vi "2-1三角函数实现(notcomplete).vi"() -> ()   [LabVIEW 2018]
uses:
  <vilib>/Analysis/3filter.llb/Filter Passband Type.ctl
  <vilib>/Analysis/3filter.llb/Butterworth Filter (DBL).vi
  <vilib>/express/express analysis/Spectral/Block/exnSpectralBlock spectral measurements peak poly.vi
  <vilib>/express/express analysis/Spectral/Block/exnSpectralBlock spectral measurements peak WFM.vi
  <vilib>/express/express analysis/Spectral/XNode/ExpressSpectralMeasurementsBlockNode.xnode
  <vilib>/measure/NI_MABase.lvlib
  <vilib>/Analysis/NI_AALBase.lvlib
  <vilib>/Analysis/NI_AALPro.lvlib
panel:
  out "载波信号":waveform(dbl)(graph)
  out "β":dbl
  in  "选项卡控件":enum32{"调制", "滤波", "解调"}(tab)
  out "频域":cluster{"f0":dbl, "df":dbl, "magnitude":dbl[]}(graph)
  out "时域":waveform(dbl)[](graph)
  out "频域":cluster{"f0":dbl, "df":dbl, "magnitude":dbl[]}(graph)
  out "时域":waveform(dbl)(graph)
  out "时域 2":waveform(dbl)(graph)
  in  "带通Butterworth滤波器":cluster{"中心频率(Hz)":dbl, "带宽(Hz)":dbl}={"中心频率(Hz)"=150000.0, "带宽(Hz)"=30000.0}
  out "BT(Hz)":dbl
  out "调制信号":waveform(dbl)(graph)
  out "采样参数（采样频率fs，采样数Ns）":cluster{dbl, dbl} {"?" format="%#_6f"; "?" format="%#_6f"}
  in  "kf(Hz/V)":dbl=50000.0
  in  "An(V)":dbl=0.02
  in  "调制信号":cluster{"fm(Hz)":dbl, "Am(V)":dbl}={"fm(Hz)"=5000.0, "Am(V)"=1.0}
  in  "载波信号":cluster{"fc(Hz)":dbl, "Ac(V)":dbl}={"fc(Hz)"=150000.0, "Ac(V)"=1.0}
  # "要显示n个周期的调制信号波形，\n则采样数Ns=n*fs/fm"
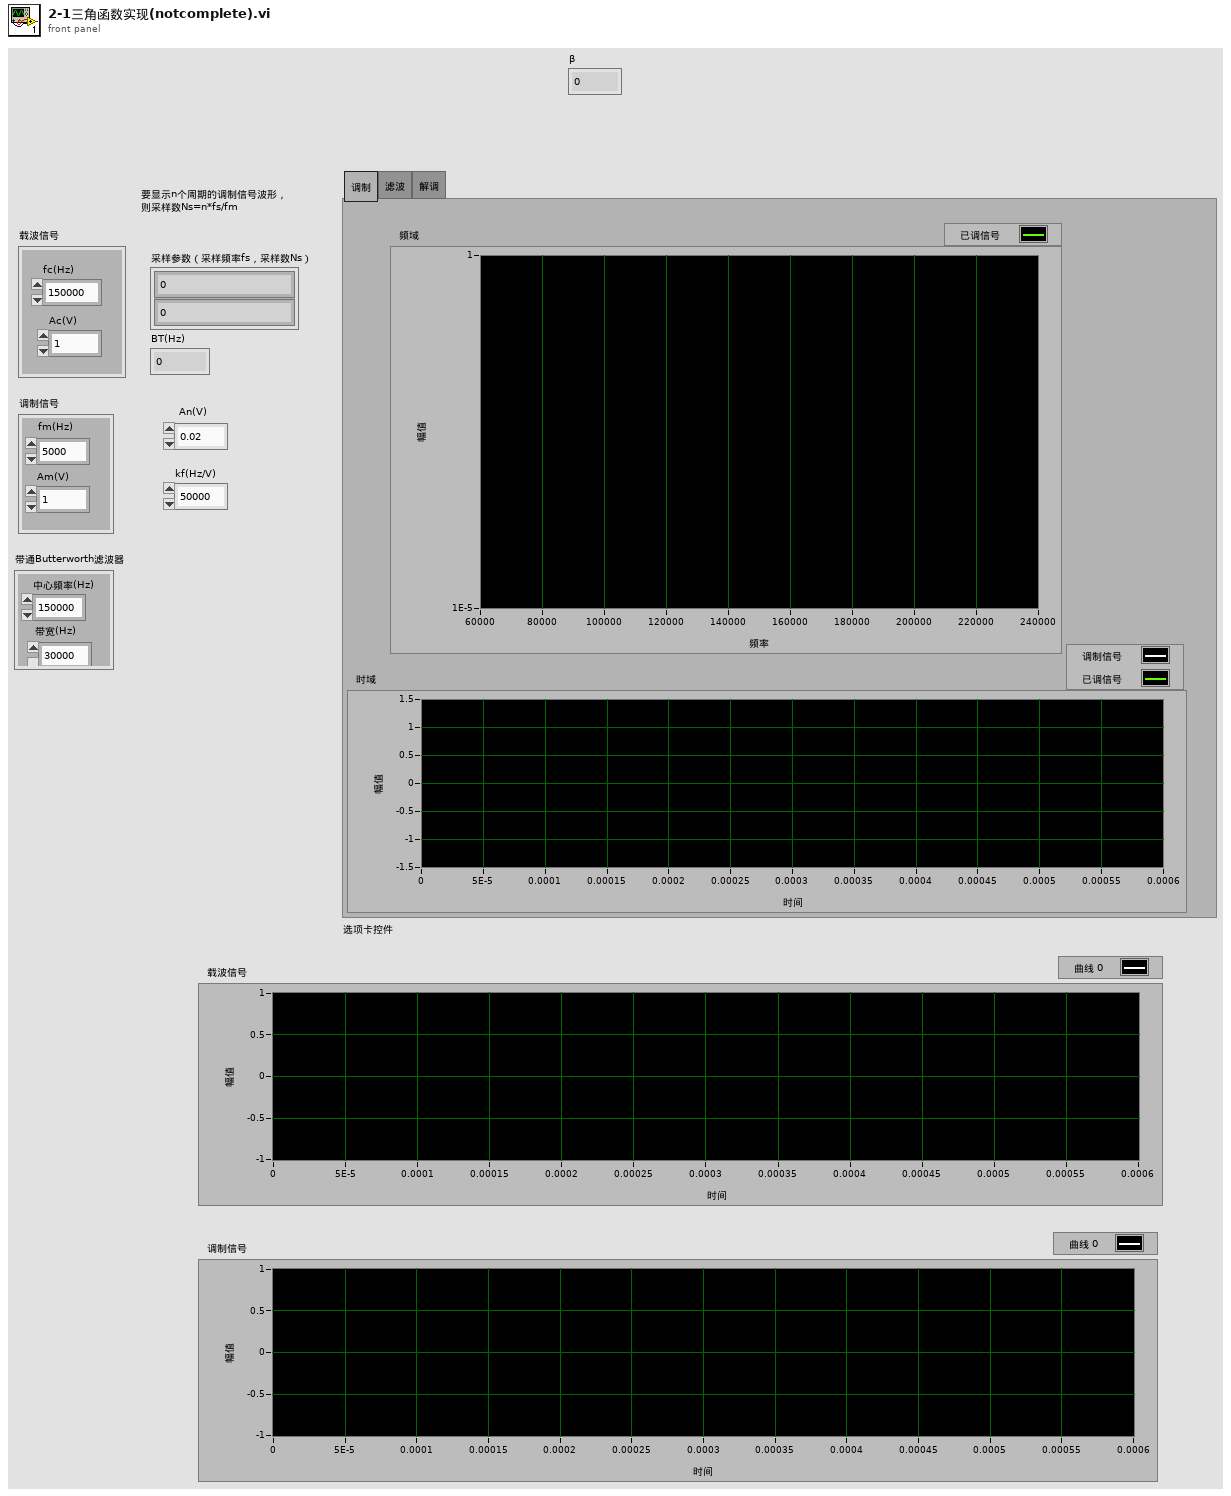
[diagram p1: front panel]
types:
  T1 = typedef "NI_AALBase.lvlib/Filter Passband Type.ctl" = enum32{"Lowpass", "Highpass", "Bandpass", "Bandstop"}
  T2 = cluster{"averaging mode":u16, "weighting mode":u16, "number of averages":u32}
  T3 = cluster{"dB On (F)":bool, "unwrap phase (F)":bool, "convert to degree (F)":bool}
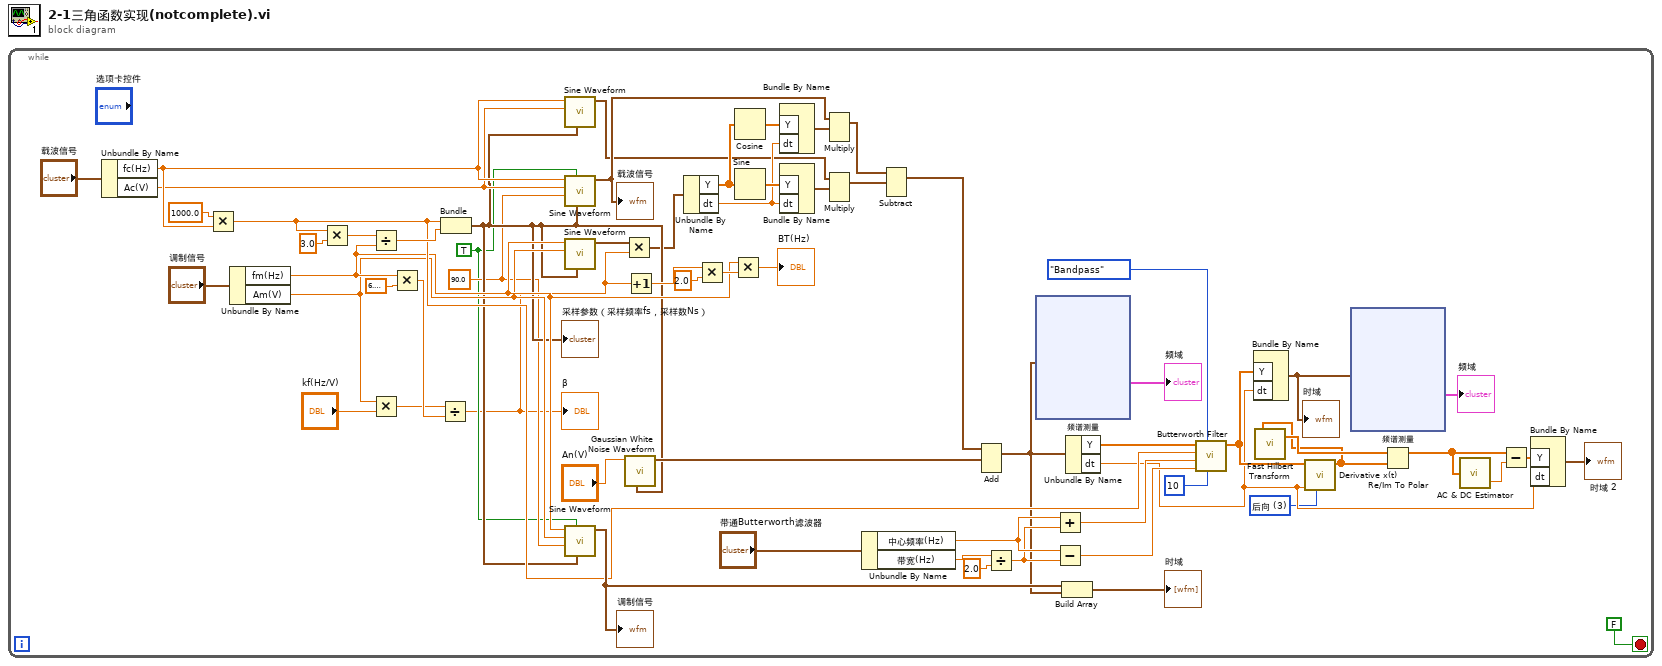
[diagram p0: block diagram]
diagram:
  n1 = while {
    stop <- FALSE stop-if-true
    w26 = u16 3 items=["二阶中心", "四阶中心", "前向", "后向"] ("method")
    w17 = 90.0 ("phase")
    w16 = TRUE ("reset signal")
    n2 = Unbundle By Name("载波信号") -> ("fc(Hz)"=w20:dbl, "Ac(V)"=w19:dbl)
    n3 = Multiply(x=1000.0, y=w20) -> (x*y=w35:dbl)
    n4 = Unbundle By Name("调制信号") -> ("fm(Hz)"=w22:dbl, "Am(V)"=w21:dbl)
    n5 = Multiply(x=w35, y=3.0) -> (x*y=w59:dbl)
    n6 = Divide(x=w59, y=w22) -> (x/y=w58:dbl)
    n7 = Multiply(x=w21, y="kf(Hz/V)") -> (x*y=w49:dbl)
    n8 = Multiply(x=w22, y=6.283185307179586) -> (x*y=w50:dbl)
    n9 = Divide(x=w49, y=w50) -> (x/y=w14:dbl)
    "β" <- w14
    n10 = Bundle(w35, w58) -> (w18:cluster{dbl, dbl})  [unwired: 1 in]
    "采样参数（采样频率fs，采样数Ns）" <- w18
    n11 = call <vilib>:"Sine Waveform.vi"("sampling info"=w18, "amplitude"=w19, "frequency"=w20) -> ("signal out"=w5:waveform(dbl))  [unwired: 7 in, 1 out]
    n12 = call <vilib>:"Sine Waveform.vi"("sampling info"=w18, "reset signal"=w16, "phase"=w17, "amplitude"=w19, "frequency"=w20) -> ("signal out"=w10:waveform(dbl))  [unwired: 5 in, 1 out]
    "载波信号" <- w10
    n13 = call <vilib>:"Sine Waveform.vi"("sampling info"=w18, "amplitude"=w21, "frequency"=w22) -> ("signal out"=w15:waveform(dbl))  [unwired: 7 in, 1 out]
    n14 = call <vilib>:"Sine Waveform.vi"("sampling info"=w18, "reset signal"=w16, "phase"=w17, "amplitude"=w21, "frequency"=w22) -> ("signal out"=w55:waveform(dbl))  [unwired: 5 in, 1 out]
    "调制信号" <- w55
    n15 = Multiply(x=w15, y=w14) -> (x*y=w13:waveform(dbl))
    n16 = call <vilib>:"Gaussian White Noise Waveform.vi"("sampling info"=w18, "standard deviation"="An(V)") -> ("signal out"=w54:waveform(dbl))  [unwired: 8 in, 1 out]
    n17 = Increment(x=w14) -> (x+1=w48:dbl)
    n18 = Unbundle By Name(w13) -> ("Y"=w9:dbl[], "dt"=w7:dbl)
    n19 = Multiply(x=w48, y=2.0) -> (x*y=w46:dbl)
    n20 = Multiply(x=w22, y=w46) -> (x*y=→"BT(Hz)":dbl)
    n21 = Cosine(x=w9) -> (cos(x)=w12:dbl[])
    n22 = Sine(x=w9) -> (sin(x)=w8:dbl[])
    n23 = Bundle By Name("Y"=w12, "dt"=w7) -> (w11:waveform(dbl))  [unwired: 1 in]
    n24 = Bundle By Name("Y"=w8, "dt"=w7) -> (w6:waveform(dbl))  [unwired: 1 in]
    n25 = Multiply(1:w11, 2:w10) -> (0:w4:waveform(dbl))  [unwired: 1 in, 1 out]
    n26 = Multiply(1:w6, 2:w5) -> (0:w3:waveform(dbl))  [unwired: 1 in, 1 out]
    n27 = Unbundle By Name("带通Butterworth滤波器") -> ("中心频率(Hz)"=w37:dbl, "带宽(Hz)"=w41:dbl)
    n28 = Subtract(1:w3, 2:w4) -> (0:w2:waveform(dbl))  [unwired: 1 in, 1 out]
    n29 = Add(1:w54, 2:w2) -> (0:w33:waveform(dbl))  [unwired: 1 in, 1 out]
    n30 = Divide(x=w41, y=2.0) -> (x/y=w36:dbl)
    n31 = xnode "频谱测量"("信号"=w33) -> ("FFT - （峰值）"=→"频域":cluster{"f0":dbl, "df":dbl, "magnitude":dbl[]})  [unwired: 1 in, 2 out]
    n32 = Add(x=w37, y=w36) -> (x+y=w39:dbl)
    n33 = Subtract(x=w37, y=w36) -> (x-y=w38:dbl)
    n34 = Build Array(w55, w33) -> (→"时域":waveform(dbl)[])
    n35 = Unbundle By Name(w33) -> ("Y"=w32:dbl[], "dt"=w28:dbl)
    n36 = call-poly <vilib>:"Butterworth Filter.vi"("order"=10, "filter type"=Filter_Passband_Type."Bandpass", "low cutoff freq: fl"=w38, "high cutoff freq: fh"=w39, "sampling freq: fs"=w35, "X"=w32) -> ("Filtered X"=w30:dbl[])  [unwired: 2 in, 1 out]
    n37 = Bundle By Name("Y"=w30, "dt"=w28) -> (w31:waveform(dbl))  [unwired: 1 in]
    "时域" <- w31
    n38 = call <vilib>:"Derivative x(t).vi"("method"=w26, "dt"=w28, "X"=w30) -> ("dX/dt"=w1:dbl[])  [unwired: 7 in, 1 out]
    n39 = call <vilib>:"Fast Hilbert Transform.vi"("X"=w1) -> ("Hilbert{X}"=w29:dbl[])  [unwired: 1 out]
    n40 = xnode "频谱测量"("信号"=w31) -> ("FFT - （峰值）"=→"频域":cluster{"f0":dbl, "df":dbl, "magnitude":dbl[]})  [unwired: 1 in, 2 out]
    n41 = Re/Im To Polar(2:w1, 3:w29) -> (1:w25:dbl[])  [unwired: 1 out]
    n42 = call <vilib>:"AC & DC Estimator.vi"("Signal (V)"=w25) -> ("DC estimate (V)"=w24:dbl)  [unwired: 1 out]
    n43 = Subtract(x=w25, y=w24) -> (x-y=w23:dbl[])
    n44 = Bundle By Name("Y"=w23, "dt"=w28) -> (→"时域 2":waveform(dbl))  [unwired: 1 in]
  }
